vi "poly_asynch_wait_start.vi"(8 "error in":errorcluster, 9 "notifier name":T1) -> (0 "error out":errorcluster, 1 "notifier name":T1, 2 "notifier":T2)   [LabVIEW 2015]
uses:
  cores/boolean_notifier.ctl
  cores/boolean_notifier_name.ctl
  poly_cast_boolean_notifier_q2n.vi
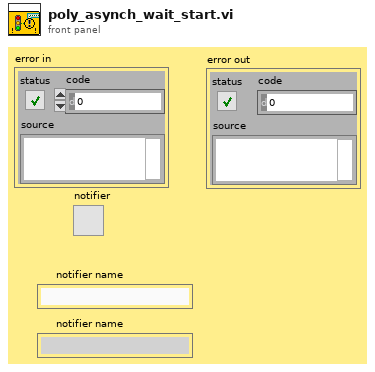
[diagram p1: front panel]
types:
  T1 = typedef "boolean_notifier_name.ctl" = string
  T2 = typedef "boolean_notifier.ctl" = refnum<k1>
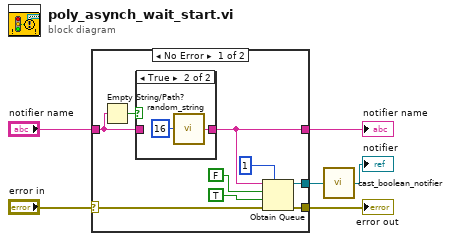
[diagram p0: block diagram]
diagram:
  n1 = case shown="No Error" "error in" {
    selector: "error in" -> [w10 w19]
    tunnel: [w9 w19] -> w6
    tunnel: "notifier name" -> [w15 _]
    tunnel: [w11 _] -> w2
    tunnel: [w13 _] -> w4
    frame No Error {
      n2 = Empty String/Path?(string/path=w15) -> (empty?=w14:bool)
      n3 = case shown="True" w14 {
        tunnel: w15 -> [w16 _]
        tunnel: [w16 w17] -> w11
        frame False {
        }
        frame True {
          n4 = call "random_string.vi"("length"=16) -> ("random string"=w17:string)  [unwired: 8 in]
        }
      }
      n5 = Obtain Queue(max queue size (-1, unlimited)=1, name (unnamed)=w11, element data type=FALSE ("data type"), create if not found? (T)=TRUE ("create new if not found"), error in (no error)=w10) -> (queue out=w13:refnum<queue>, error out=w9:errorcluster)  [unwired: 1 out]
    }
    frame Error {
    }
  }
  "error out" <- w6
  "notifier name" <- w2
  n6 = call-poly "cast_boolean_notifier.vi"("boolean queue"=w4) -> ("boolean notifier"=→"notifier":T2)  [unwired: 8 in]
